vi "ServoControl.vi"() -> ()   [LabVIEW 2016]
uses:
  <vilib>/rvi/interface/nirviCloseFPGA/nirviCloseFPGA.xnode
  <vilib>/rvi/interface/nirviMethod/nirviMethod.xnode
  <vilib>/rvi/interface/nirviReadWriteControl/nirviReadWriteControl.xnode
  <vilib>/rvi/interface/nirviOpenFPGA/nirviOpenFPGA.xnode
  FPGA Bitfiles/VisionTest_FPGATarget_FPGAMain_jZlYpbXtgx0.lvbitx
  <vilib>/FPGAPlugInAG/myRIO-1900/niLvFpga_Close_myRIO-1900.vi
  <vilib>/FPGAPlugInAG/myRIO-1900/niLvFpga_Open_myRIO-1900.vi
  <vilib>/FPGAPlugInAG/myRIO-1900/niLvFpga_Run_myRIO-1900.vi
  NiFpgaLv.dll
  <vilib>/Utility/error.llb/Error Cluster From Error Code.vi
  <vilib>/rvi/errors/niLvFpgaAdjustHostInterfaceError.vi
panel:
  in  "Servo2HighTime":u32(slide) scale=320.0..1900.0
  in  "stop":bool
  in  "Servo1HighTime":u32(slide) scale=320.0..1900.0
  # "Workable servo high times\n\n320uS - 1900uS\n\nApprox 100 degrees"
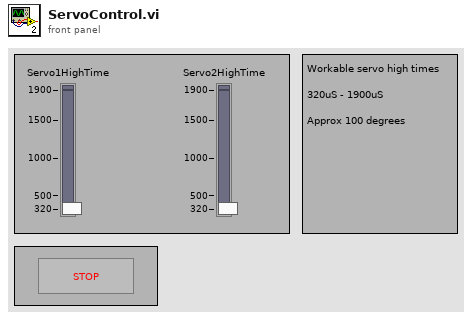
[diagram p1: front panel]
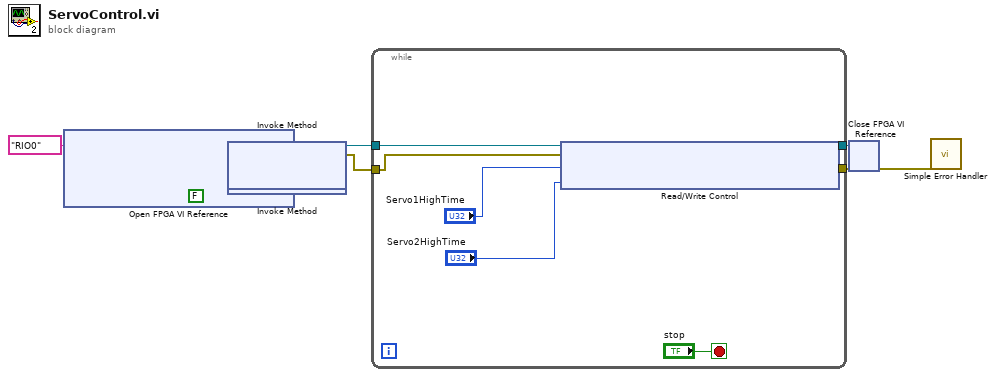
[diagram p0: block diagram]
diagram:
  n1 = xnode "Open FPGA VI Reference"("resource name"=tag "RIO0") -> ("FPGA VI Reference Out"=w4:refnum<k20>, "error out"=w3:errorcluster)  [unwired: 1 in]
  n2 = xnode "Invoke Method"("FPGA VI Reference In"=w4, "error in"=w3, "Wait Until Done (F)"=FALSE) -> ("FPGA VI Reference Out"=w6:refnum<k20>, "error out"=w5:errorcluster)
  n3 = xnode "Invoke Method"() -> ()  [unwired: 3 in, 2 out]
  n4 = while {
    tunnel: w6 -> [w15]
    tunnel: [w12] -> w9
    tunnel: [w13] -> w8
    tunnel: w5 -> [w14]
    stop <- "stop" stop-if-true
    n5 = xnode "Read/Write Control"("FPGA VI Reference In"=w15, "error in"=w14, "Servo1HighTime"="Servo1HighTime", "Servo2HighTime"="Servo2HighTime") -> ("FPGA VI Reference Out"=w12:refnum<k20>, "error out"=w13:errorcluster)
  }
  n6 = xnode "Close FPGA VI Reference"("FPGA VI Reference In"=w9, "error in"=w8) -> ("error out"=w7:errorcluster)
  n7 = call <vilib>:"Simple Error Handler.vi"("error in (no error)"=w7) -> ()  [unwired: 4 in, 5 out]
